vi "Horizontal Query.vi"(8 "error in":errorcluster, 11 "Instrument Handle In":i32) -> (0 "error out":errorcluster, 1 "Sample Time":dbl, 2 "Sample Points":u32, 3 "Instrument Handle Out":i32, 4 "Offset Time":dbl)   [LabVIEW 2020, in "ZTScopeM.lvlib"]
doc: "Query the horizontal and timebase settings."
uses:
  ZTScopeM.lvlib
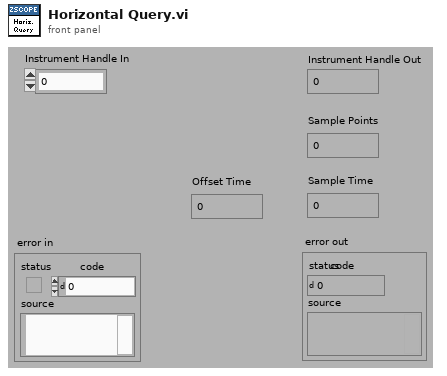
[diagram p1: front panel]
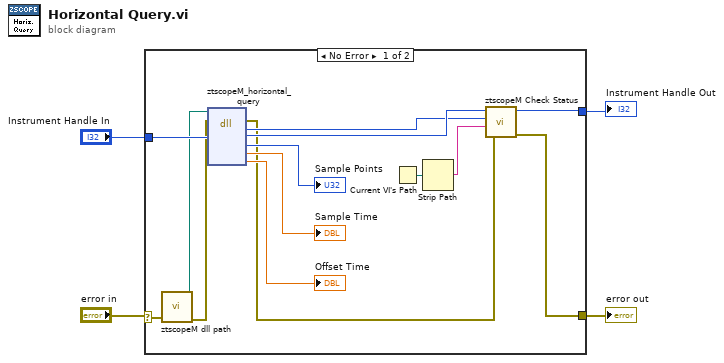
[diagram p0: block diagram]
diagram:
  n1 = case shown="No Error" "error in" {
    selector: "error in" -> [w8 w20]
    tunnel: [w10 w20] -> w1
    tunnel: "Instrument Handle In" -> [w18 w19]
    tunnel: [w9 w19] -> w3
    frame No Error {
      n2 = call "ztscopeM dll path.vi"("error in (no error)"=w8) -> ("error out"=w6:errorcluster, "<instrument>.dll path"=w7:path)  [unwired: 9 in]
      n3 = dll-call lib="C:/Program Files (x86)/National Instruments/LabVIEW 2013/instr.lib/ztscopem/ztscopeM.dll" fn="ztscopeM_horizontal_query"(path in=w7, error in=w6, "instrumentHandle"=w18) -> (error out=w5:errorcluster, w11:i32, "instrumentHandle"=w12:i32, "samplePoints"=→"Sample Points":u32, "sampleTime"=→"Sample Time":dbl, "offsetTime"=→"Offset Time":dbl)  [unwired: 4 in, 1 out]
      n4 = Current VI's Path() -> (path=w14:path)
      n5 = Strip Path(path=w14) -> (name=w13:string)  [unwired: 1 out]
      n6 = call "ztscopeM Check Status.vi"("error in"=w5, "name of VI"=w13, "status (return code)"=w11, "instrument handle in"=w12) -> ("error out"=w10:errorcluster, "instrument handle out"=w9:i32)  [unwired: 2 in]
    }
    frame Error {
    }
  }
  "Instrument Handle Out" <- w3
  "error out" <- w1
